vi "PID_controller_08.vi"() -> ()   [LabVIEW 2011]
uses:
  <vilib>/Platform/TimedLoop/XDataNode/nitl_modes.ctl
  <vilib>/Platform/TimedLoop/XDataNode/timing_clust.ctl
  <vilib>/Platform/TimedLoop/XDataNode/wakeup.ctl
  <vilib>/Platform/TimedLoop/XDataNode/XDataNode.xnode
  <vilib>/Platform/TimedLoop/XDataNode/XDNodeRunTimeDep.lvlib
panel:
  out "Setpoint":string
  out "Angle (deg)":string
  in  "Ks":dbl
  out "dt(s)":dbl
  out "windup error":dbl
  out "tPrev":dbl
  out "target value":dbl
  out "error(t-t0)":cluster{dbl, "Value":dbl}[](array[cluster])
  out "error":dbl
  out "tStart(s)":dbl
  out "S00":dbl
  out "S10":dbl
  out "S20":dbl
  out "S11":dbl
  out "S01":dbl
  out "weight":dbl[](array[numeric])
  in  "# of points to watch":i32
  in  "tSmooth(s)":dbl=-1.0
  out "t0":dbl
  out "error(t)":cluster{dbl, "Value":dbl}[](array[cluster])
  out "error out":errorcluster
  out "first":bool=TRUE
  out "P (torr)":string
  out "XY Graph":cluster{dbl, "Value":dbl}[](graph)
  out "current value":dbl
  in  "stop":bool
  in  "Period (s)":dbl
  out "dValue":dbl
  out "derivative":dbl
  out "integral":dbl
  out "Current angle (deg)":dbl
  in  "Kd":dbl
  in  "Ki":dbl
  in  "Kp":dbl
  out "Current P (torr)":dbl
  in  "Set Point (torr)":dbl
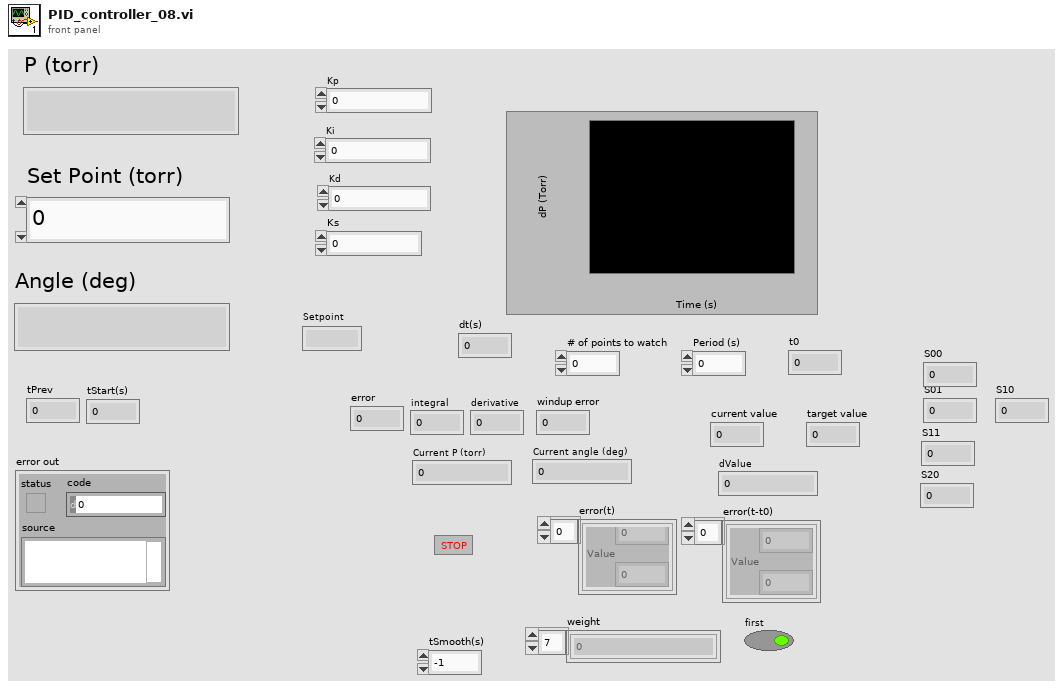
[diagram p1: front panel]
types:
  T1 = typedef "XDNodeRunTimeDep.lvlib/nitl_modes.ctl" = enum32{"No Change", "Process missed periods, maintain original phase", "Discard missed periods, maintain original phase", "Process missed periods, ignore original phase", "Discard missed periods, ignore original phase"}
  T2 = typedef "XDNodeRunTimeDep.lvlib/timing_clust.ctl" = cluster{"Expected End [f-1]":u64, "Actual End [f-1]":u64, "Finished Late? [f-1]":bool, "Expected End [i-1]":u64, "Actual End [i-1]":u64, "Finished Late? [i-1]":bool, "Expected Start [i]":u64, "Actual Start [i]":u64, "Expected Start [f]":u64, "Actual Start [f]":u64, "Source Name":string, "Structure Name":string, "Period":i64, "Deadline":i64, "Offset":i64, "Start":i64, "Priority":i32, "Timeout":i32, "Mode":T1, "Wakeup Reason":T3, "Error":errorcluster, "Source Type":string, "Secondary Source Type":string, "Global End Time":u64, "Global Start Time":u64, "Frame Duration":u64, "Iteration Duration":u64, "Assigned CPU":i32, "I/O Scan Engine Mode":u32}
  T3 = typedef "XDNodeRunTimeDep.lvlib/wakeup.ctl" = enum32{"Normal", "Aborted", "Asynchronous wakeup", "Timing source error", "Timed loop error", "Timeout"}
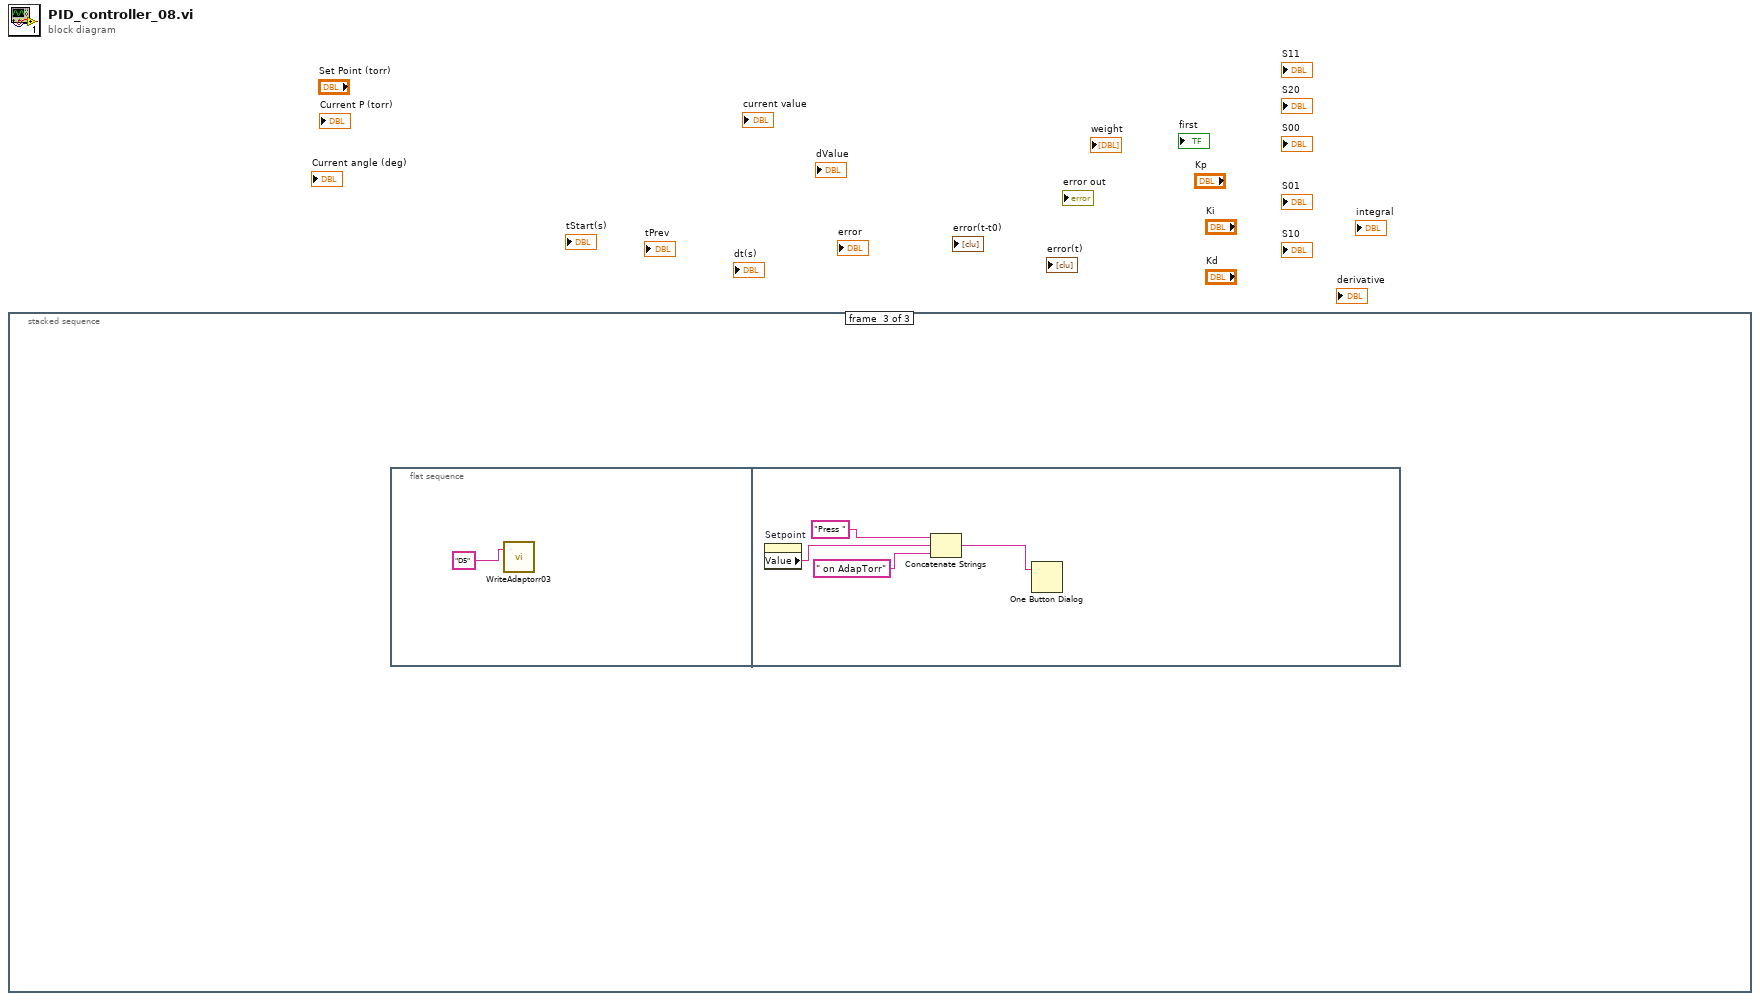
[diagram p0: block diagram]
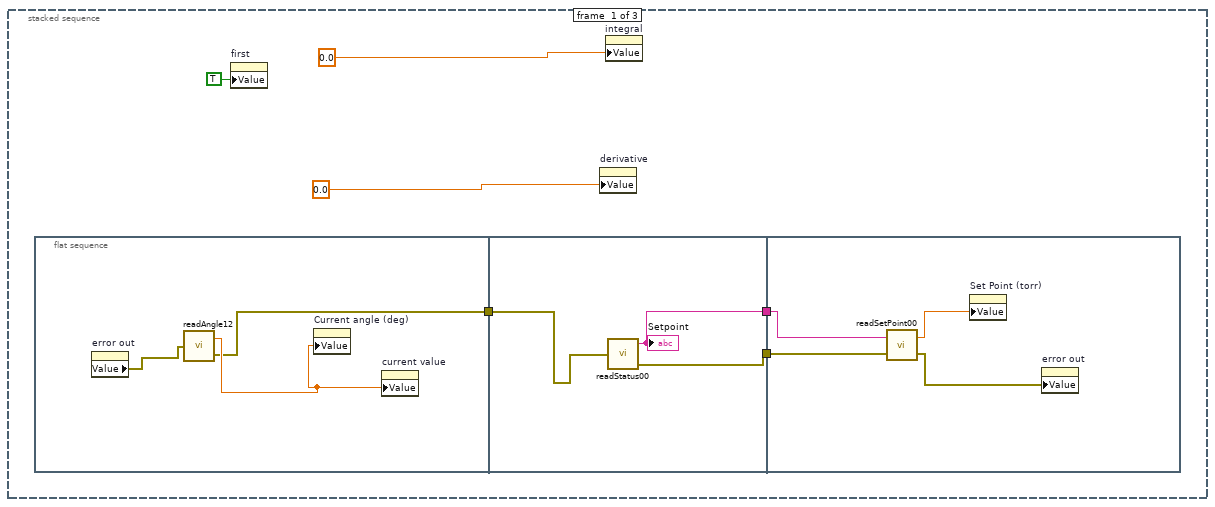
[diagram p2: hidden frame]
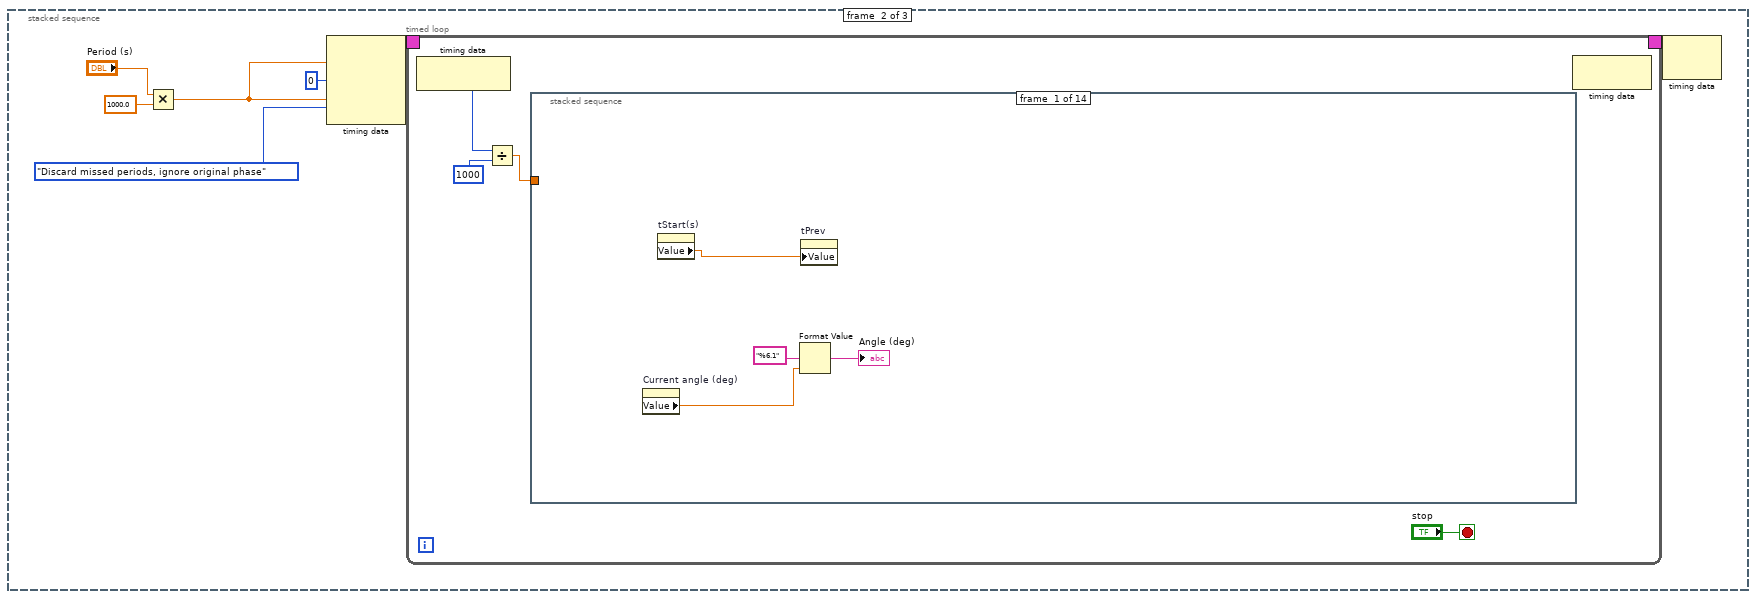
[diagram p3: hidden frame]
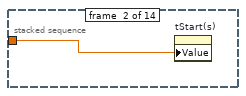
[diagram p4: hidden frame]
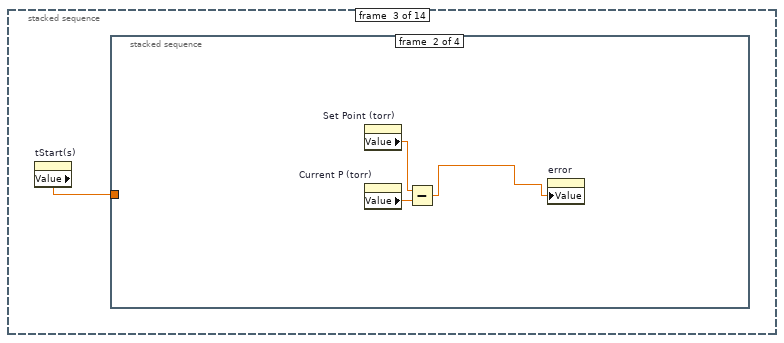
[diagram p5: hidden frame]
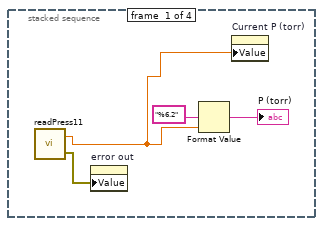
[diagram p6: hidden frame]
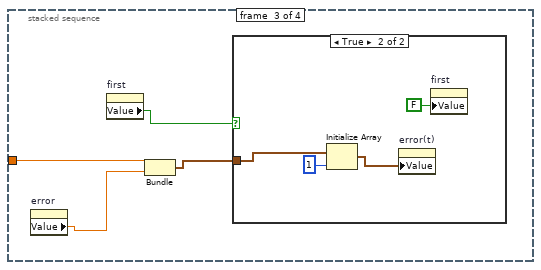
[diagram p7: hidden frame]
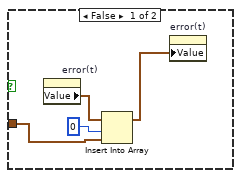
[diagram p8: hidden frame]
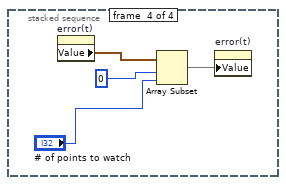
[diagram p9: hidden frame]
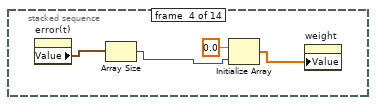
[diagram p10: hidden frame]
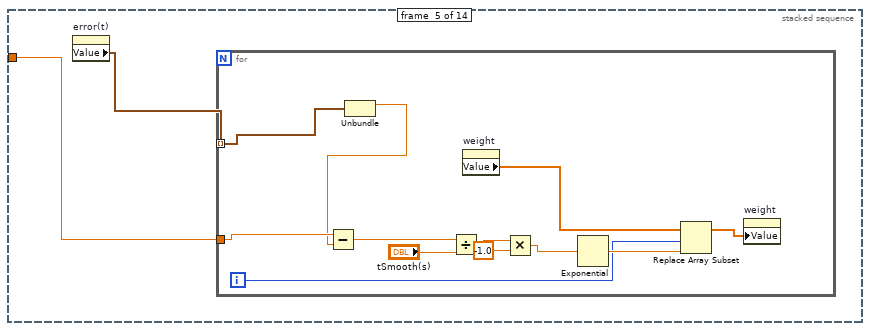
[diagram p11: hidden frame]
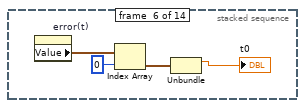
[diagram p12: hidden frame]
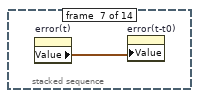
[diagram p13: hidden frame]
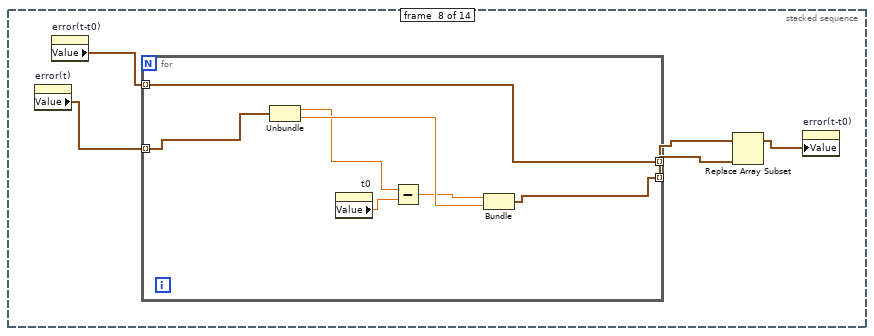
[diagram p14: hidden frame]
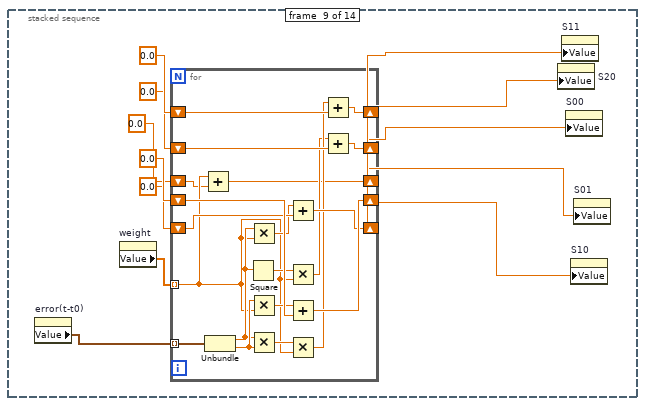
[diagram p15: hidden frame]
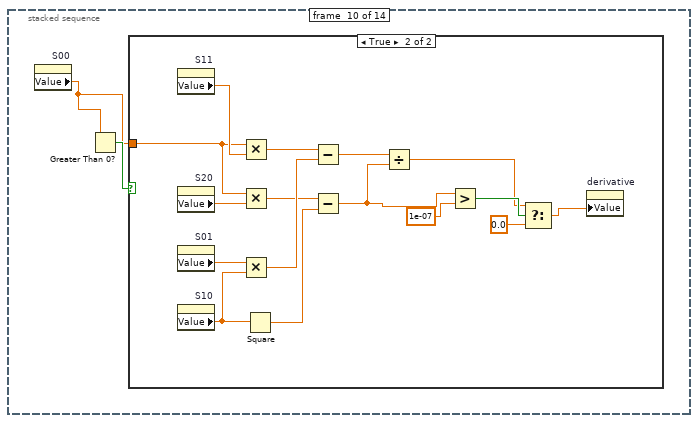
[diagram p16: hidden frame]
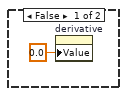
[diagram p17: hidden frame]
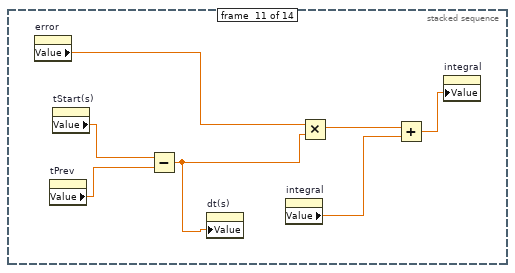
[diagram p18: hidden frame]
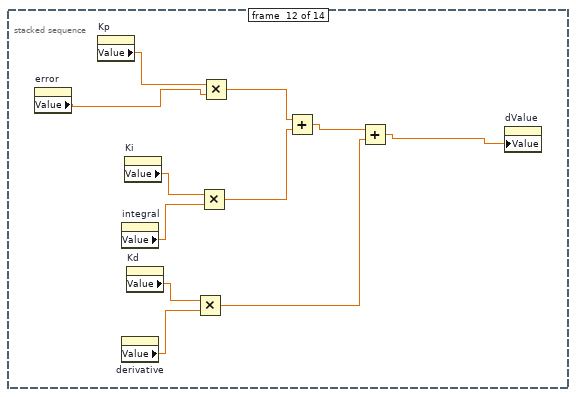
[diagram p19: hidden frame]
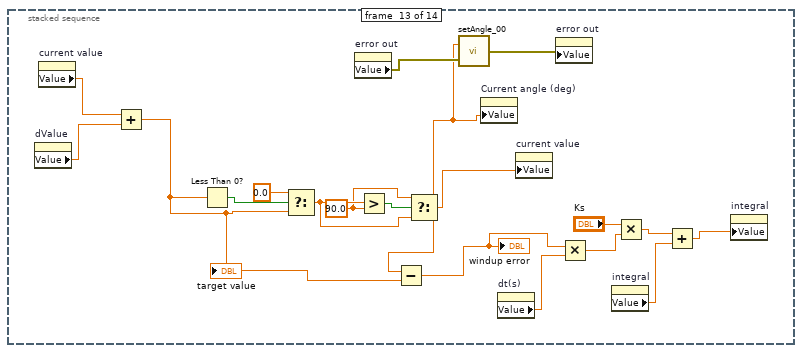
[diagram p20: hidden frame]
diagram:
  n1 = stacked-sequence {
    frame #0 {
      n2 = flat-sequence {
        tunnel: [w7] -> w1
        tunnel: [w12] -> w3
        tunnel: [w11] -> w2
        tunnel: w1 -> [w10]
        tunnel: w3 -> [w16]
        tunnel: w2 -> [w15]
        frame #0 {
          n3 = property on="error out" class="Clust (strict)"() -> ("Value"=w9:errorcluster)  [unwired: 2 in, 2 out]
          n4 = call "readAngle12.vi"("error in"=w9) -> ("angle"=w8:dbl, "error out"=w7:errorcluster)
          n5 = property on="Current angle (deg)" class="DigNum (strict)"("Value"=w8) -> ()  [unwired: 2 in, 2 out]
          n6 = property on="current value" class="DigNum (strict)"("Value"=w8) -> ()  [unwired: 2 in, 2 out]
        }
        frame #1 {
          n7 = call "readStatus00.vi"("error in"=w10) -> ("Setpoint"=w12:string, "error out"=w11:errorcluster)  [unwired: 1 out]
          "Setpoint" <- w12
        }
        frame #2 {
          n8 = call "readSetPoint00.vi"("error in"=w15, "Setpoint"=w16) -> ("error out"=w14:errorcluster, "P"=w13:dbl)
          n9 = property on="Set Point (torr)" class="DigNum (strict)"("Value"=w13) -> ()  [unwired: 2 in, 2 out]
          n10 = property on="error out" class="Clust (strict)"("Value"=w14) -> ()  [unwired: 2 in, 2 out]
        }
      }
      n11 = property on="first" class="Bool (strict)"("Value"=TRUE ("first")) -> ()  [unwired: 2 in, 2 out]
      n12 = property on="derivative" class="DigNum (strict)"("Value"=0.0 ("derivative")) -> ()  [unwired: 2 in, 2 out]
      n13 = property on="integral" class="DigNum (strict)"("Value"=0.0 ("integral")) -> ()  [unwired: 2 in, 2 out]
    }
    frame #1 {
      n14 = Multiply(x="Period (s)", y=1000.0) -> (x*y=w18:dbl)
      n15 = node-c288(w18, i64 0 ("Offset"), w18, nitl_modes."Discard missed periods, ignore original phase" ("Mode")) -> (w23:T2)
      n16 = timed-loop {
        timing: w23 -> [_]
        timing-out: [_] -> w22
        stop <- "stop" stop-if-true
        n17 = node-c288() -> (w24:i64)  [unwired: 1 in]
        n18 = Divide(x=w24, y=i64 1000) -> (x/y=w25:dbl)
        n19 = stacked-sequence {
          tunnel: w25 -> [_ w32 _ _ w61 _ _ _ _ _ _ _ _ _]
          frame #0 {
            n20 = property on="Current angle (deg)" class="DigNum (strict)"() -> ("Value"=w28:dbl)  [unwired: 2 in, 2 out]
            n21 = property on="tStart(s)" class="DigNum (strict)"() -> ("Value"=w31:dbl)  [unwired: 2 in, 2 out]
            n22 = Format Value(format string="%6.1", value (0)=w28) -> (output string=→"Angle (deg)":string)  [unwired: 1 in]
            n23 = property on="tPrev" class="DigNum (strict)"("Value"=w31) -> ()  [unwired: 2 in, 2 out]
          }
          frame #1 {
            n24 = property on="tStart(s)" class="DigNum (strict)"("Value"=w32) -> ()  [unwired: 2 in, 2 out]
          }
          frame #2 {
            n25 = property on="tStart(s)" class="DigNum (strict)"() -> ("Value"=w33:dbl)  [unwired: 2 in, 2 out]
            n26 = stacked-sequence {
              tunnel: w33 -> [_ _ w43 _]
              frame #0 {
                n27 = call "readPress11.vi"() -> ("P"=w35:dbl, "error out"=w34:errorcluster)  [unwired: 1 in]
                n28 = property on="error out" class="Clust (strict)"("Value"=w34) -> ()  [unwired: 2 in, 2 out]
                n29 = Format Value(format string="%6.2", value (0)=w35) -> (output string=→"P (torr)":string)  [unwired: 1 in]
                n30 = property on="Current P (torr)" class="DigNum (strict)"("Value"=w35) -> ()  [unwired: 2 in, 2 out]
              }
              frame #1 {
                n31 = property on="Set Point (torr)" class="DigNum (strict)"() -> ("Value"=w39:dbl)  [unwired: 2 in, 2 out]
                n32 = property on="Current P (torr)" class="DigNum (strict)"() -> ("Value"=w40:dbl)  [unwired: 2 in, 2 out]
                n33 = Subtract(x=w39, y=w40) -> (x-y=w38:dbl)
                n34 = property on="error" class="DigNum (strict)"("Value"=w38) -> ()  [unwired: 2 in, 2 out]
              }
              frame #2 {
                n35 = property on="error" class="DigNum (strict)"() -> ("Value"=w41:dbl)  [unwired: 2 in, 2 out]
                n36 = property on="first" class="Bool (strict)"() -> ("Value"=w44:bool)  [unwired: 2 in, 2 out]
                n37 = Bundle("Value"=w43, "Value"=w41) -> (w42:cluster{"Value":dbl, "Value":dbl})  [unwired: 1 in]
                n38 = case shown="True" w44 {
                  tunnel: w42 -> [w46 w51]
                  frame False {
                    n39 = property on="error(t)" class="Arr (strict)"() -> ("Value"=w47:cluster{dbl, "Value":dbl}[])  [unwired: 2 in, 2 out]
                    n40 = Insert Into Array(array=w47, index=0, new element=w46) -> (w45:cluster{dbl, "Value":dbl}[])
                    n41 = property on="error(t)" class="Arr (strict)"("Value"=w45) -> ()  [unwired: 2 in, 2 out]
                  }
                  frame True {
                    n42 = Initialize Array(w51, 1 ("dimension size")) -> (w49:cluster{"Value":dbl, "Value":dbl}[])
                    n43 = property on="error(t)" class="Arr (strict)"("Value"=w49) -> ()  [unwired: 2 in, 2 out]
                    n44 = property on="first" class="Bool (strict)"("Value"=FALSE ("first")) -> ()  [unwired: 2 in, 2 out]
                  }
                }
              }
              frame #3 {
                n45 = property on="error(t)" class="Arr (strict)"() -> ("Value"=w54:cluster{dbl, "Value":dbl}[])  [unwired: 2 in, 2 out]
                n46 = Array Subset(array=w54, index=0, length="# of points to watch") -> (w56:cluster{dbl, "Value":dbl}[])
                n47 = property on="error(t)" class="Arr (strict)"("Value"=w56) -> ()  [unwired: 2 in, 2 out]
              }
            }
          }
          frame #3 {
            n48 = property on="error(t)" class="Arr (strict)"() -> ("Value"=w60:cluster{dbl, "Value":dbl}[])  [unwired: 2 in, 2 out]
            n49 = Array Size(array=w60) -> (size(s)=w58:i32)
            n50 = Initialize Array(0.0 ("element"), w58) -> (w57:dbl[])
            n51 = property on="weight" class="Arr (strict)"("Value"=w57) -> ()  [unwired: 2 in, 2 out]
          }
          frame #4 {
            n52 = property on="error(t)" class="Arr (strict)"() -> ("Value"=w62:cluster{dbl, "Value":dbl}[])  [unwired: 2 in, 2 out]
            n53 = for {
              tunnel: w62 -> [w74] mode=indexing
              tunnel: w61 -> [w73]
              i -> [w69]
              n54 = Unbundle(w74) -> (w72:dbl)  [unwired: 1 out]
              n55 = Subtract(x=w73, y=w72) -> (x-y=w67:dbl)
              n56 = Divide(x=w67, y="tSmooth(s)") -> (x/y=w65:dbl)
              n57 = property on="weight" class="Arr (strict)"() -> ("Value"=w70:dbl[])  [unwired: 2 in, 2 out]
              n58 = Multiply(x=w65, y=-1.0) -> (x*y=w63:dbl)
              n59 = Exponential(1:w63) -> (0:w71:dbl)
              n60 = Replace Array Subset(array=w70, new element=w71, index=w69) -> (w68:dbl[])
              n61 = property on="weight" class="Arr (strict)"("Value"=w68) -> ()  [unwired: 2 in, 2 out]
            }
          }
          frame #5 {
            n62 = property on="error(t)" class="Arr (strict)"() -> ("Value"=w78:cluster{dbl, "Value":dbl}[])  [unwired: 2 in, 2 out]
            n63 = Index Array(array=w78, index=0) -> (element=w76:cluster{dbl, "Value":dbl})
            n64 = Unbundle(w76) -> (→"t0":dbl)  [unwired: 1 out]
          }
          frame #6 {
            n65 = property on="error(t)" class="Arr (strict)"() -> ("Value"=w79:cluster{dbl, "Value":dbl}[])  [unwired: 2 in, 2 out]
            n66 = property on="error(t-t0)" class="Arr (strict)"("Value"=w79) -> ()  [unwired: 2 in, 2 out]
          }
          frame #7 {
            n67 = property on="error(t)" class="Arr (strict)"() -> ("Value"=w84:cluster{dbl, "Value":dbl}[])  [unwired: 2 in, 2 out]
            n68 = property on="error(t-t0)" class="Arr (strict)"() -> ("Value"=w82:cluster{dbl, "Value":dbl}[])  [unwired: 2 in, 2 out]
            n69 = for {
              tunnel: w84 -> [w87] mode=indexing
              tunnel: [w86] -> w83 mode=indexing
              tunnel: w82 -> [w85] mode=indexing
              tunnel: [w85] -> w81 mode=indexing
              n70 = Unbundle(w87) -> (w88:dbl, "Value"=w90:dbl)
              n71 = property on="t0" class="DigNum (strict)"() -> ("Value"=w91:dbl)  [unwired: 2 in, 2 out]
              n72 = Subtract(x=w88, y=w91) -> (x-y=w89:dbl)
              n73 = Bundle(w89, "Value"=w90) -> (w86:cluster{dbl, "Value":dbl})  [unwired: 1 in]
            }
            n74 = Replace Array Subset(array=w81, new element=w83) -> (w80:cluster{dbl, "Value":dbl}[])  [unwired: 1 in]
            n75 = property on="error(t-t0)" class="Arr (strict)"("Value"=w80) -> ()  [unwired: 2 in, 2 out]
          }
          frame #8 {
            n76 = property on="error(t-t0)" class="Arr (strict)"() -> ("Value"=w92:cluster{dbl, "Value":dbl}[])  [unwired: 2 in, 2 out]
            n77 = property on="weight" class="Arr (strict)"() -> ("Value"=w99:dbl[])  [unwired: 2 in, 2 out]
            n78 = for {
              tunnel: w92 -> [w119] mode=indexing
              shift-right: [w120] -> w94
              shift-left: 0.0 -> [w123]
              shift-right: [w116] -> w97
              shift-left: 0.0 -> [w122]
              shift-right: [w115] -> w96
              shift-left: 0.0 -> [w121]
              shift-right: [w117] -> w93
              shift-left: 0.0 -> [w118]
              tunnel: w99 -> [w106] mode=indexing
              shift-right: [w104] -> w95
              shift-left: 0.0 -> [w105]
              n79 = Add(x=w106, y=w105) -> (x+y=w104:dbl)
              n80 = Unbundle(w119) -> (w108:dbl, "Value"=w114:dbl)
              n81 = Square(x=w108) -> (x^2=w110:dbl)
              n82 = Multiply(x=w108, y=w106) -> (x*y=w107:dbl)
              n83 = Multiply(x=w114, y=w106) -> (x*y=w113:dbl)
              n84 = Multiply(x=w108, y=w114) -> (x*y=w112:dbl)
              n85 = Add(x=w107, y=w118) -> (x+y=w117:dbl)
              n86 = Multiply(x=w110, y=w106) -> (x*y=w109:dbl)
              n87 = Add(x=w113, y=w123) -> (x+y=w120:dbl)
              n88 = Multiply(x=w112, y=w106) -> (x*y=w111:dbl)
              n89 = Add(x=w111, y=w122) -> (x+y=w116:dbl)
              n90 = Add(x=w109, y=w121) -> (x+y=w115:dbl)
            }
            n91 = property on="S20" class="DigNum (strict)"("Value"=w96) -> ()  [unwired: 2 in, 2 out]
            n92 = property on="S11" class="DigNum (strict)"("Value"=w97) -> ()  [unwired: 2 in, 2 out]
            n93 = property on="S00" class="DigNum (strict)"("Value"=w95) -> ()  [unwired: 2 in, 2 out]
            n94 = property on="S10" class="DigNum (strict)"("Value"=w93) -> ()  [unwired: 2 in, 2 out]
            n95 = property on="S01" class="DigNum (strict)"("Value"=w94) -> ()  [unwired: 2 in, 2 out]
          }
          frame #9 {
            n96 = property on="S00" class="DigNum (strict)"() -> ("Value"=w124:dbl)  [unwired: 2 in, 2 out]
            n97 = Greater Than 0?(x=w124) -> (x > 0?=w125:bool)
            n98 = case shown="True" w125 {
              tunnel: w124 -> [_ w134]
              frame False {
                n99 = property on="derivative" class="DigNum (strict)"("Value"=0.0 ("derivative")) -> ()  [unwired: 2 in, 2 out]
              }
              frame True {
                n100 = property on="S11" class="DigNum (strict)"() -> ("Value"=w136:dbl)  [unwired: 2 in, 2 out]
                n101 = property on="S20" class="DigNum (strict)"() -> ("Value"=w135:dbl)  [unwired: 2 in, 2 out]
                n102 = property on="S01" class="DigNum (strict)"() -> ("Value"=w133:dbl)  [unwired: 2 in, 2 out]
                n103 = property on="S10" class="DigNum (strict)"() -> ("Value"=w137:dbl)  [unwired: 2 in, 2 out]
                n104 = Multiply(x=w134, y=w136) -> (x*y=w142:dbl)
                n105 = Multiply(x=w134, y=w135) -> (x*y=w140:dbl)
                n106 = Multiply(x=w133, y=w137) -> (x*y=w141:dbl)
                n107 = Square(x=w137) -> (x^2=w139:dbl)
                n108 = Subtract(x=w142, y=w141) -> (x-y=w138:dbl)
                n109 = Subtract(x=w140, y=w139) -> (x-y=w132:dbl)
                n110 = Divide(x=w138, y=w132) -> (x/y=w128:dbl)
                n111 = Greater?(x=w132, y=1e-07) -> (0:w130:bool)
                n112 = Select(t=w128, s=w130, f=0.0) -> (s? t:f=w129:dbl)
                n113 = property on="derivative" class="DigNum (strict)"("Value"=w129) -> ()  [unwired: 2 in, 2 out]
              }
            }
          }
          frame #10 {
            n114 = property on="error" class="DigNum (strict)"() -> ("Value"=w147:dbl)  [unwired: 2 in, 2 out]
            n115 = property on="tPrev" class="DigNum (strict)"() -> ("Value"=w148:dbl)  [unwired: 2 in, 2 out]
            n116 = property on="tStart(s)" class="DigNum (strict)"() -> ("Value"=w149:dbl)  [unwired: 2 in, 2 out]
            n117 = Subtract(x=w149, y=w148) -> (x-y=w143:dbl)
            n118 = property on="dt(s)" class="DigNum (strict)"("Value"=w143) -> ()  [unwired: 2 in, 2 out]
            n119 = property on="integral" class="DigNum (strict)"() -> ("Value"=w145:dbl)  [unwired: 2 in, 2 out]
            n120 = Multiply(x=w147, y=w143) -> (x*y=w146:dbl)
            n121 = Add(x=w146, y=w145) -> (x+y=w144:dbl)
            n122 = property on="integral" class="DigNum (strict)"("Value"=w144) -> ()  [unwired: 2 in, 2 out]
          }
          frame #11 {
            n123 = property on="error" class="DigNum (strict)"() -> ("Value"=w150:dbl)  [unwired: 2 in, 2 out]
            n124 = property on="Kp" class="DigNum (strict)"() -> ("Value"=w160:dbl)  [unwired: 2 in, 2 out]
            n125 = property on="integral" class="DigNum (strict)"() -> ("Value"=w158:dbl)  [unwired: 2 in, 2 out]
            n126 = property on="derivative" class="DigNum (strict)"() -> ("Value"=w156:dbl)  [unwired: 2 in, 2 out]
            n127 = property on="Ki" class="DigNum (strict)"() -> ("Value"=w159:dbl)  [unwired: 2 in, 2 out]
            n128 = property on="Kd" class="DigNum (strict)"() -> ("Value"=w157:dbl)  [unwired: 2 in, 2 out]
            n129 = Multiply(x=w157, y=w156) -> (x*y=w153:dbl)
            n130 = Multiply(x=w159, y=w158) -> (x*y=w154:dbl)
            n131 = Multiply(x=w160, y=w150) -> (x*y=w155:dbl)
            n132 = Add(x=w155, y=w154) -> (x+y=w152:dbl)
            n133 = Add(x=w152, y=w153) -> (x+y=w151:dbl)
            n134 = property on="dValue" class="DigNum (strict)"("Value"=w151) -> ()  [unwired: 2 in, 2 out]
          }
          frame #12 {
            w170 = 90.0 ("y")
            n135 = property on="dValue" class="DigNum (strict)"() -> ("Value"=w177:dbl)  [unwired: 2 in, 2 out]
            n136 = property on="current value" class="DigNum (strict)"() -> ("Value"=w178:dbl)  [unwired: 2 in, 2 out]
            n137 = Add(x=w178, y=w177) -> (x+y=w161:dbl)
            "target value" <- w161
            n138 = Less Than 0?(x=w161) -> (x < 0?=w174:bool)
            n139 = Select(t=0.0, s=w174, f=w161) -> (s? t:f=w171:dbl)
            n140 = property on="error out" class="Clust (strict)"() -> ("Value"=w176:errorcluster)  [unwired: 2 in, 2 out]
            n141 = Greater?(x=w171, y=w170) -> (0:w172:bool)
            n142 = Select(t=w170, s=w172, f=w171) -> (s? t:f=w162:dbl)
            n143 = Subtract(x=w162, y=w161) -> (x-y=w169:dbl)
            "windup error" <- w169
            n144 = call "setAngle_00.vi"("error in (no error)"=w176, "Angle (deg)"=w162) -> ("error out"=w175:errorcluster)
            n145 = property on="Current angle (deg)" class="DigNum (strict)"("Value"=w162) -> ()  [unwired: 2 in, 2 out]
            n146 = property on="dt(s)" class="DigNum (strict)"() -> ("Value"=w168:dbl)  [unwired: 2 in, 2 out]
            n147 = property on="current value" class="DigNum (strict)"("Value"=w162) -> ()  [unwired: 2 in, 2 out]
            n148 = property on="error out" class="Clust (strict)"("Value"=w175) -> ()  [unwired: 2 in, 2 out]
            n149 = Multiply(x=w169, y=w168) -> (x*y=w167:dbl)
            n150 = property on="integral" class="DigNum (strict)"() -> ("Value"=w164:dbl)  [unwired: 2 in, 2 out]
            n151 = Multiply(x="Ks", y=w167) -> (x*y=w165:dbl)
            n152 = Add(x=w165, y=w164) -> (x+y=w163:dbl)
            n153 = property on="integral" class="DigNum (strict)"("Value"=w163) -> ()  [unwired: 2 in, 2 out]
          }
          frame #13 {
            n154 = property on="error(t-t0)" class="Arr (strict)"() -> ("Value"=→"XY Graph":cluster{dbl, "Value":dbl}[])  [unwired: 2 in, 2 out]
          }
        }
        n155 = node-c288() -> ()  [unwired: 1 in, 1 out]
      }
      n156 = node-c288(w22) -> ()  [unwired: 1 out]
    }
    frame #2 {
      n157 = flat-sequence {
        frame #0 {
          n158 = call "WriteAdaptorr03.vi"("string to write"="D5") -> ()  [unwired: 1 in, 1 out]
        }
        frame #1 {
          n159 = property on="Setpoint" class="Str"() -> ("Value"=w192:string)  [unwired: 2 in, 2 out]
          n160 = Concatenate Strings("Press ", w192, " on AdapTorr") -> (w191:string)
          n161 = One Button Dialog(message=w191) -> ()  [unwired: 1 in, 1 out]
        }
      }
    }
  }
